vi "Plotter_UI_Plot_Samples_FGV.vi"(7 "Initialize ?":bool, 8 "error in (no error)":errorcluster, 9 "Parameter name":string, 10 "Time (ms)":dbl, 11 "Value":dbl) -> (0 "error out":errorcluster, 3 "Samples & timestamp":T1(array[cluster]))   [LabVIEW 2017]
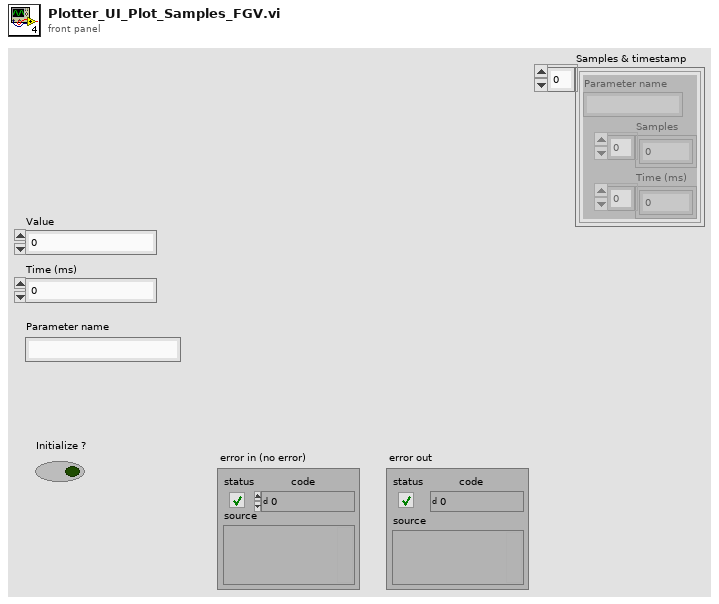
[diagram p1: front panel]
types:
  T1 = cluster{"Parameter name":string, "Samples":dbl[], "Time (ms)":dbl[]}[]
  T2 = cluster{"Parameter name":string, "Samples":dbl[], "Time (ms)":dbl[]}
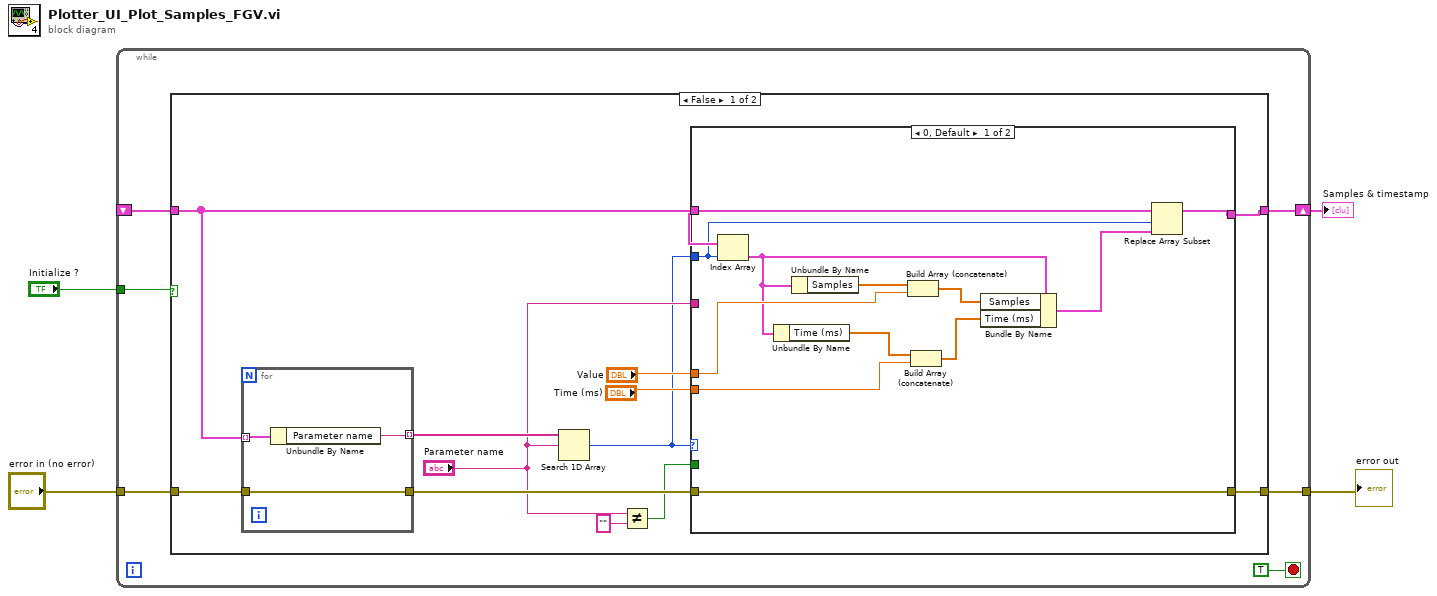
[diagram p0: block diagram]
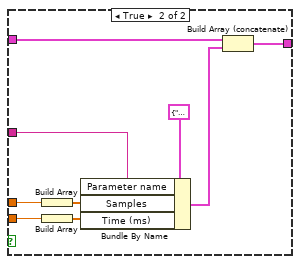
[diagram p3: hidden frame]
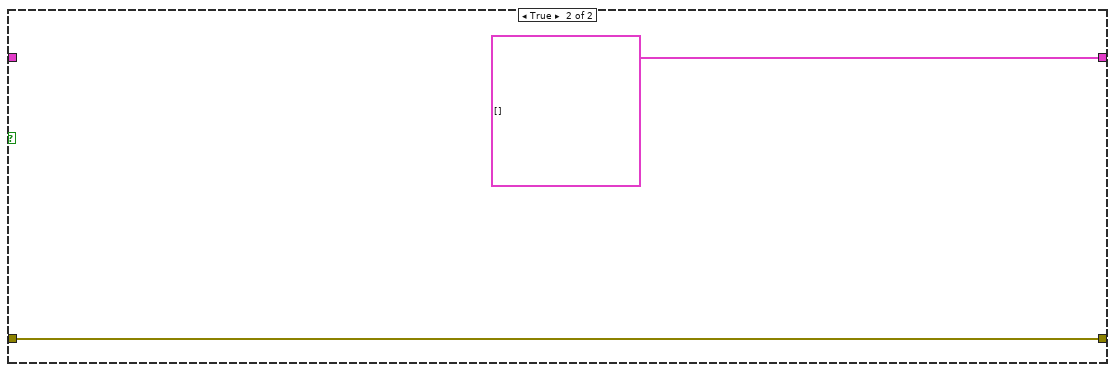
[diagram p4: hidden frame]
diagram:
  n1 = while {
    tunnel: "Initialize ?" -> [w10]
    tunnel: "error in (no error)" -> [w7]
    tunnel: [w6] -> w2
    shift-right: [w9] -> w1
    shift-left: _ -> [w5]
    stop <- TRUE stop-if-true
    n2 = case shown="False" w10 {
      tunnel: [w15 T1 []] -> w9
      tunnel: w7 -> [w22 w55]
      tunnel: [w19 w55] -> w6
      tunnel: w5 -> [w18 _]
      frame False {
        n3 = for {
          tunnel: w22 -> [w52]
          tunnel: w18 -> [w54] mode=indexing
          tunnel: [w53] -> w21 mode=indexing
          tunnel: [w52] -> w20
          n4 = Unbundle By Name(w54) -> ("Parameter name"=w53:string)
        }
        n5 = Search 1D Array(1D array=w21, element="Parameter name") -> (index of element=w11:i32)  [unwired: 1 in]
        n6 = Not Equal?(x="Parameter name", y="") -> (x != y?=w12:bool)
        n7 = case shown="0, Default" w11 {
          tunnel: w20 -> [w24 w41]
          tunnel: [w24 w41] -> w19
          tunnel: w18 -> [w27 w40]
          tunnel: "Parameter name" -> [_ w39]
          tunnel: "Value" -> [w33 w38]
          tunnel: "Time (ms)" -> [w31 w37]
          tunnel: [w26 w36] -> w15
          tunnel: w12 -> [_ w35]
          tunnel: w11 -> [w23 _]
          frame 0, Default {
            n8 = Index Array(array=w27, index=w23) -> (element=w30:T2)
            n9 = Unbundle By Name(w30) -> ("Time (ms)"=w32:dbl[])
            n10 = Unbundle By Name(w30) -> ("Samples"=w34:dbl[])
            n11 = Build Array (concatenate)(w34, w33) -> (w29:dbl[])
            n12 = Build Array (concatenate)(w32, w31) -> (w28:dbl[])
            n13 = Bundle By Name(cluster=w30, "Samples"=w29, "Time (ms)"=w28) -> (w25:T2)
            n14 = Replace Array Subset(array=w27, new element=w25, index=w23) -> (w26:T1)
          }
          frame -1 {
            n15 = case shown="False" w35 {
              tunnel: w40 -> [w42 w51]
              tunnel: w39 -> [_ w49]
              tunnel: w38 -> [_ w48]
              tunnel: w37 -> [_ w46]
              tunnel: [w42 w43] -> w36
              frame False {
              }
              frame True {
                n16 = Build Array(w48) -> (w47:dbl[])
                n17 = Build Array(w46) -> (w45:dbl[])
                n18 = Bundle By Name(cluster=T2 {"Parameter name"="", "Samples"=[], "Time (ms)"=[]}, "Parameter name"=w49, "Samples"=w47, "Time (ms)"=w45) -> (w44:T2)
                n19 = Build Array (concatenate)(w51, w44) -> (w43:T1)
              }
            }
          }
        }
      }
      frame True {
      }
    }
  }
  "error out" <- w2
  "Samples & timestamp" <- w1
